vi "UI.vi"(0 "GUI":refnum<class "GUI Sensor Lib.lvclass">, 5 "error in (no error)":errorcluster) -> (14 "reference out":refnum<class "GUI Sensor Lib.lvclass">, 19 "error out":errorcluster)   [LabVIEW 2019, in "GUI Sensor Lib.lvclass"]
uses:
  GUI Sensor Lib.lvclass
  D:/GIT H4000/H4000/src/GUI_class/GUI.lvclass
  TypeDef/GUI AI Ranges.ctl
  TypeDef/AI_Data.ctl
  TypeDef/AI Statistics Data.ctl
  GUI_class/GUI.lvclass/GUI.ctl
  TypeDef/Scale Data.ctl
  TypeDef/AI_Data_Array.ctl
  SV_Wrap/SharedVariableWrapper.lvclass/SharedVariableWrapper.ctl
  TypeDef/CalibrationData.ctl
  TypeDef/GUI Setting Channel.ctl
  MessageAMC_class/MessageAMC.lvclass
  D:/GIT H4000/H4000/src/MessageInterface_class/MessageInterface.lvclass
  <vilib>/Utility/miscctls.llb/LVStringsAndValuesArrayTypeDef_U16.ctl
  3f3c674f-4e90-49b5-a3bd-8b60e7823021.vi
  423febd4-7e95-46d1-90fe-d3c0b325c46b.vi
  73d7f925-78bb-4209-8c05-97525a648225.vi
  GUI_class/Set Win State.vi
  GUI_class/protected/GetSheredData.vi
  3f3c674f-4e90-49b5-a3bd-8b60e7823021.vi/a0a37fc8-e280-45ed-9300-29015878ae2c.vi
  SV_Wrap/Write Var Info.vi
  SV_Wrap/Read Var Info.vi
  423febd4-7e95-46d1-90fe-d3c0b325c46b.vi/498ba6c8-7b3f-45b0-8939-59de8baaa4e4.vi
  SV_Wrap/Read connection str.vi
  <userlib>/_OpenG.lib/time/time.llb/Tick Count (ms)__ogtk.vi
  GUI_class/GUI.lvclass
  MessageInterface_class/MessageInterface.lvclass
  SV_Wrap/SharedVariableWrapper.lvclass
panel:
  out "element":T1 {"Stat Data"."scl mean 1Hz" format="%0.2f"; "Stat Data"."raw mean 1Hz" format="%0.2f"; "Stat Data"."scl mean" format="%0.2f"; "Stat Data"."raw mean" format="%0.2f"}
  in  "channel indx":T3(radio)
  in  "Edit scale":bool
  in  "Scales":i32(listbox) caption="Шкалы"
  in  "Remove scl":bool
  in  "Add scl":bool
  in  "channels":cluster{"name":string, "scale indx":u16}[](array[cluster])
  out "Gauge":dbl(knob) scale=0.0..10.0
  in  "manual enter raw":bool caption="Ввод  вручную"
  in  "Scaled":dbl caption="Калиброванное  значение"
  in  "Raw":dbl caption="Необработанное значение"
  in  "data":i32(listbox)
  in  "Remove":bool
  in  "Add":bool
  out "XY Graph - Dark":cluster{"X":dbl[], "Y":dbl[]}(graph) caption="Шкала"
  in  "AI Ranges":T4
  # "SCALED"
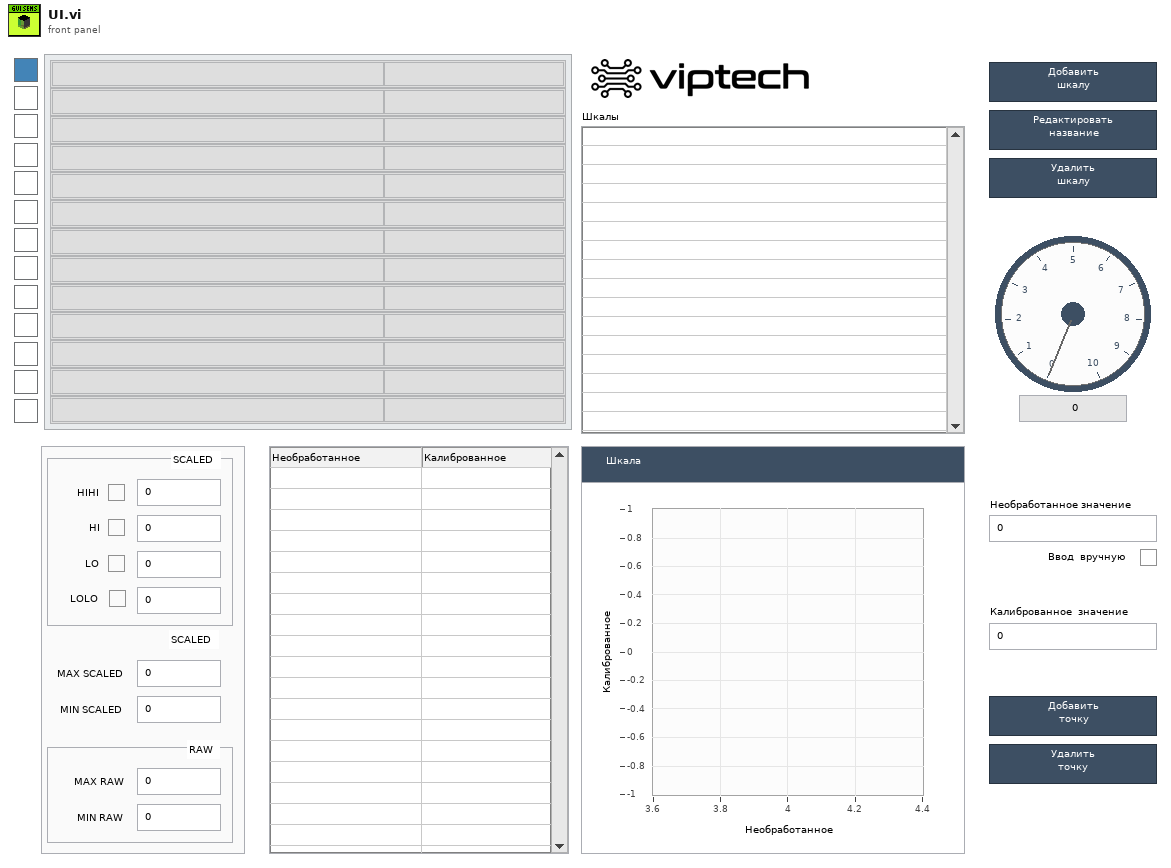
[diagram p1: front panel]
types:
  T1 = typedef "AI_Data.ctl" = cluster{"Stat Data":T2, "OutOfRangeMax":bool, "OutOfRangeMin":bool, "HIHI":bool, "HI":bool, "LO":bool, "LOLO":bool}
  T2 = typedef "AI Statistics Data.ctl" = cluster{"raw mean":dbl, "scl mean":dbl, "raw mean 1Hz":dbl, "scl mean 1Hz":dbl}
  T3 = enum32{"Item 0", "Item 1", "Item 2", "Item 3", "Item 4", "Item 5", "Item 6", "Item 7", "Item 8", "Item 9", "Item 10", "Item 11", "Item 12"}
  T4 = typedef "GUI AI Ranges.ctl" = cluster{"HI":bool, "HIHI":bool, "LO":bool, "LOLO":bool, "HIHI VAL":dbl, "HI VAL":dbl, "LO VAL":dbl, "LOLO VAL":dbl, "MAX RAW":dbl, "MIN RAW":dbl, "MAX SCALED":dbl, "MIN SCALED":dbl}
  T5 = typedef "Scale Data.ctl" = cluster{"index":i32, "Name":string, "X":dbl[], "Y":dbl[]}
  T6 = typedef "AI_Data_Array.ctl" = T1[]
  T7 = enum32{"Invalid", "Standard", "Closed", "Hidden", "Minimized", "Maximized"}
  T8 = enum32{"invalid app kind", "Development System", "Run Time System", "Student Edition", "Embedded LabVIEW", "Evaluation", "Custom"}
  T9 = typedef "CalibrationData.ctl" = cluster{"Channels":T10[], "Scales":T5[]}
  T10 = typedef "GUI Setting Channel.ctl" = cluster{"Name":string, "AI Ranges":T4, "ScaleIndex":u32}
  T11 = typedef "LVStringsAndValuesArrayTypeDef_U16.ctl" = cluster{"String":string, "Value":u16}[]
  T12 = cluster{"Core":cluster{"Current VI Reference":refnum<vi>, "Close Panel on Exit?":bool}, "CalibrationData":T9, "VAR":string, "valid data":bool, "amc":refnum<class "MessageAMC.lvclass">, "channel indx":enum32{"Item 0", "Item 1", "Item 2", "Item 3", "Item 4", "Item 5", "Item 6", "Item 7", "Item 8", "Item 9", "Item 10", "Item 11", "Item 12"}, "Scales ref":refnum<vi>, "scale indx ref":refnum<vi>}
  T13 = cluster{"Current VI Reference":refnum<vi>, "Close Panel on Exit?":bool}
  T14 = typedef "SharedVariableWrapper.lvclass/Config.ctl" = cluster{"connection str":string, "timeout":dbl, "ip":string}
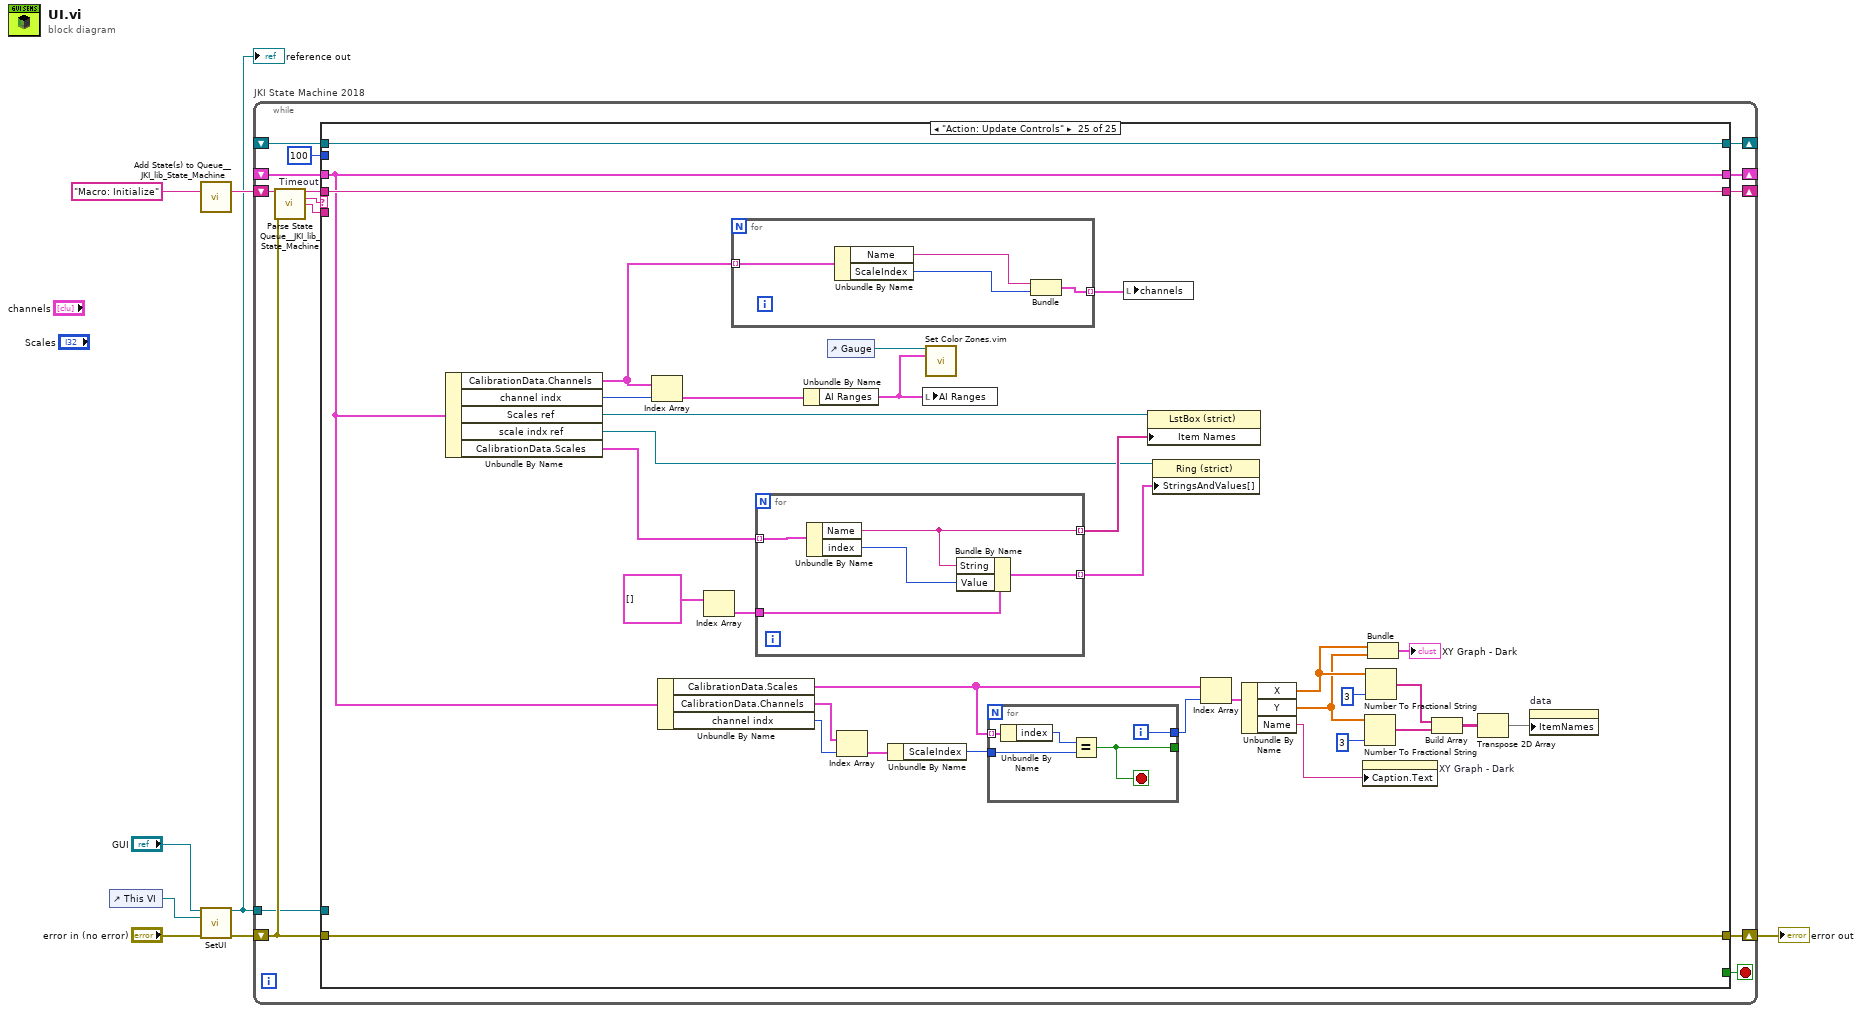
[diagram p0: block diagram]
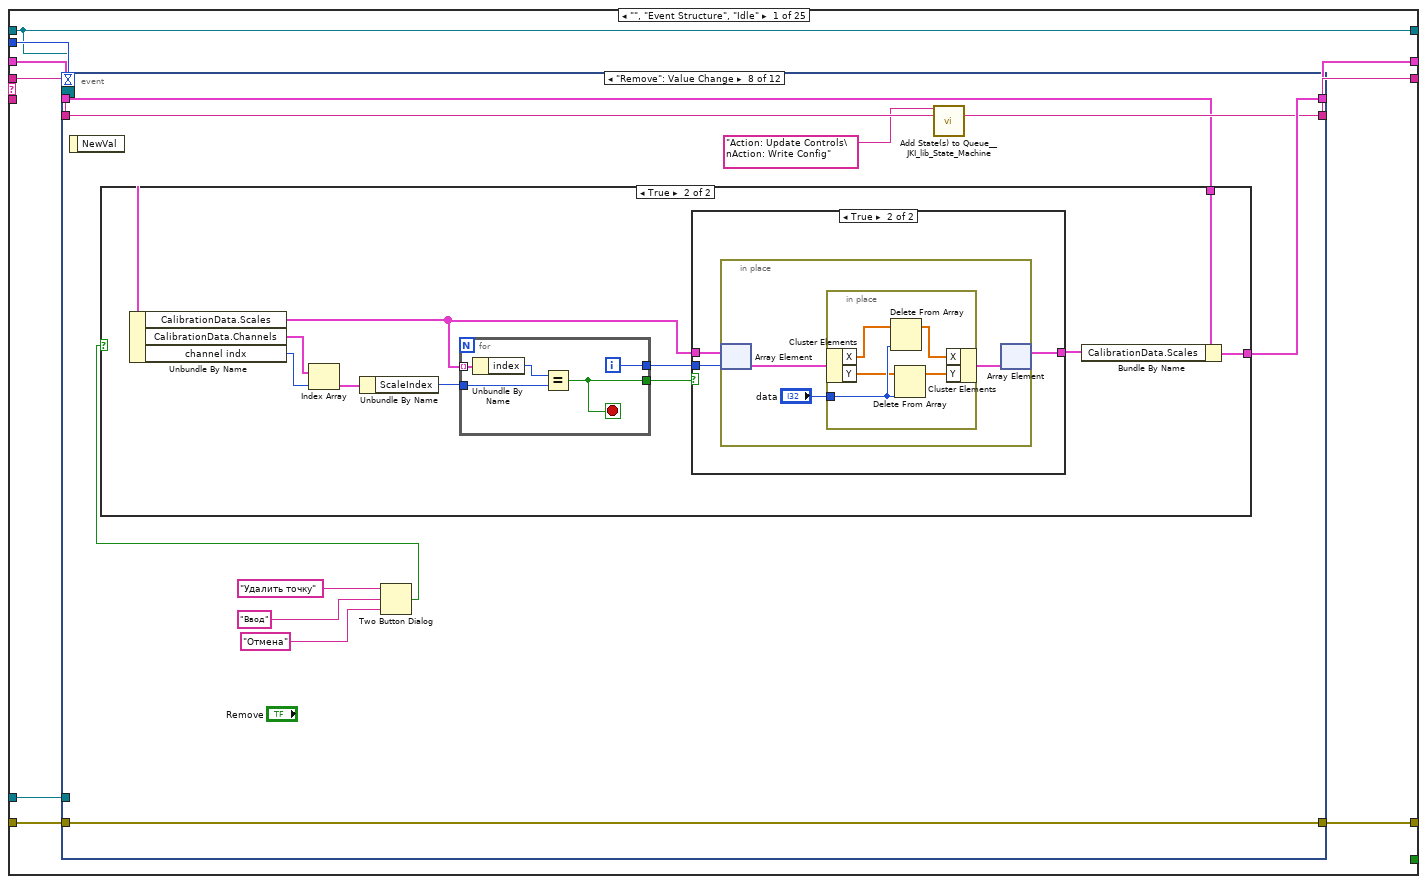
[diagram p2: hidden frame]
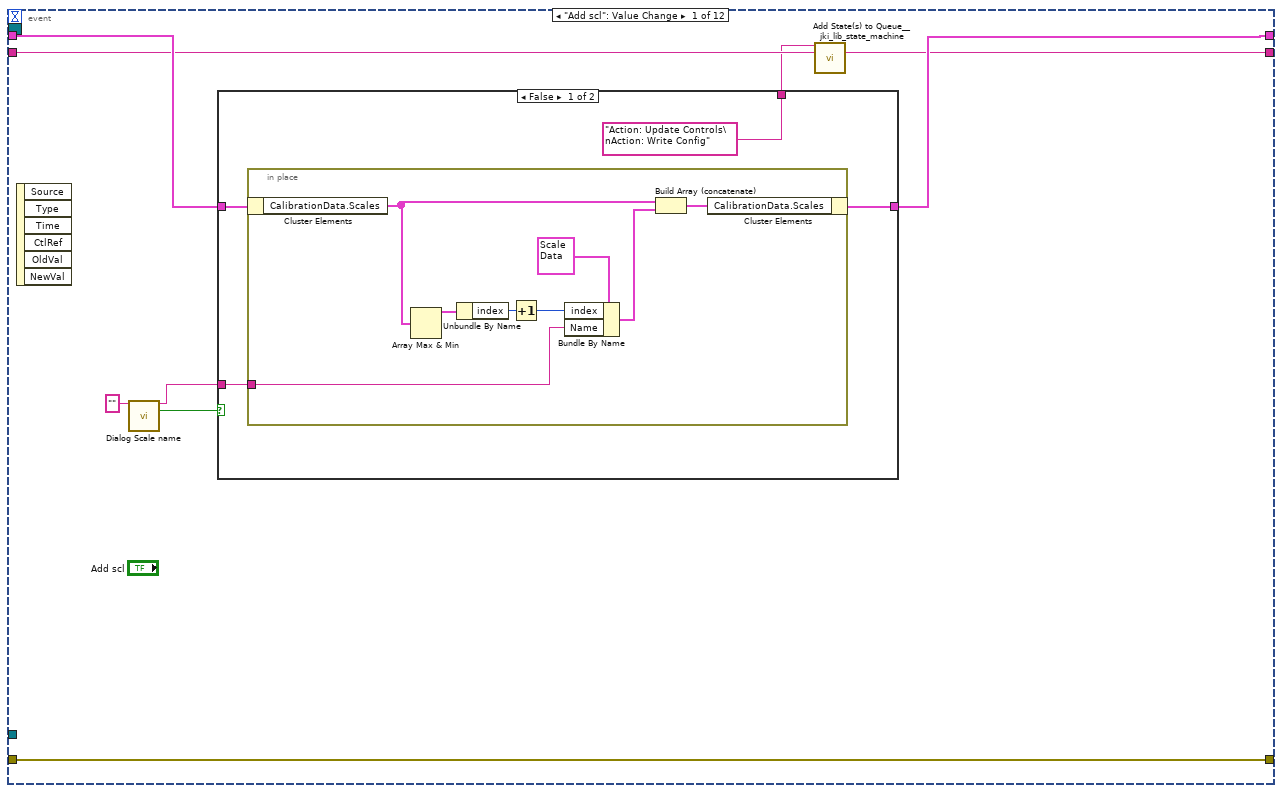
[diagram p3: hidden frame]
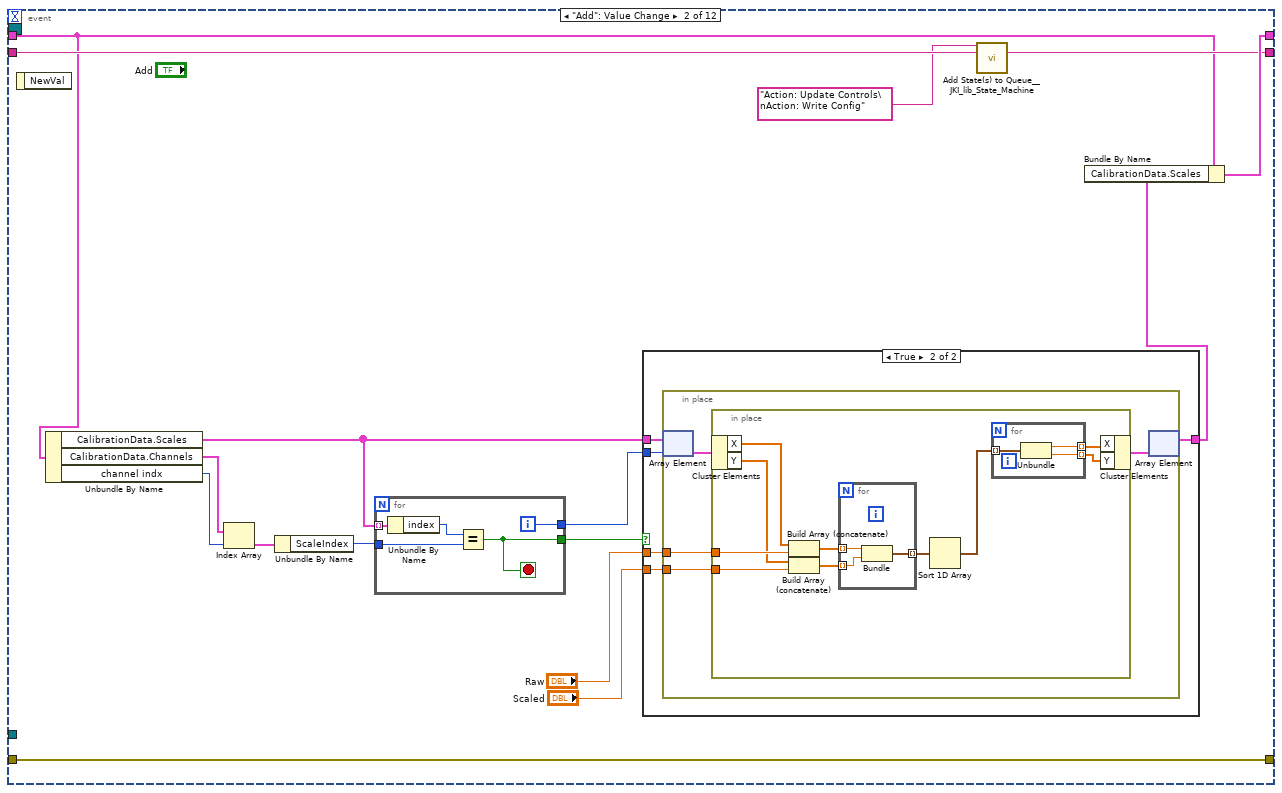
[diagram p5: hidden frame]
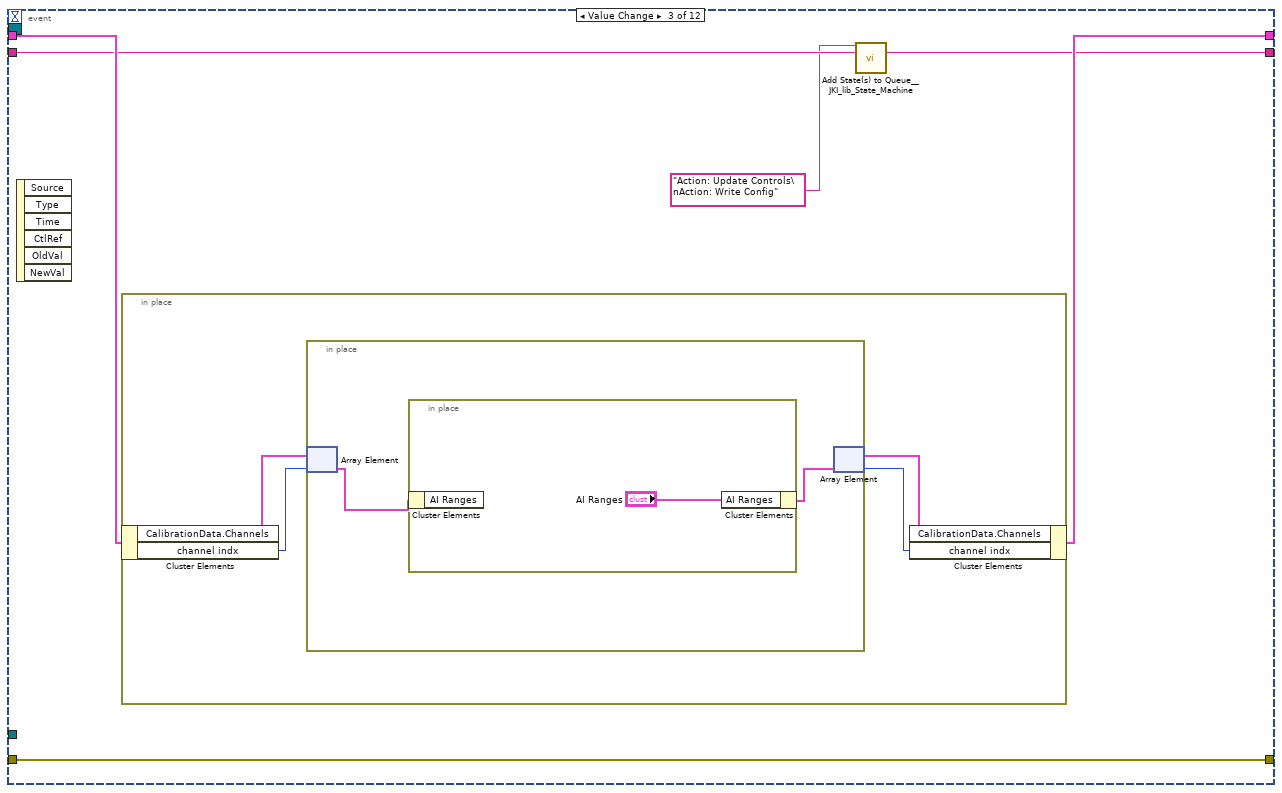
[diagram p7: hidden frame]
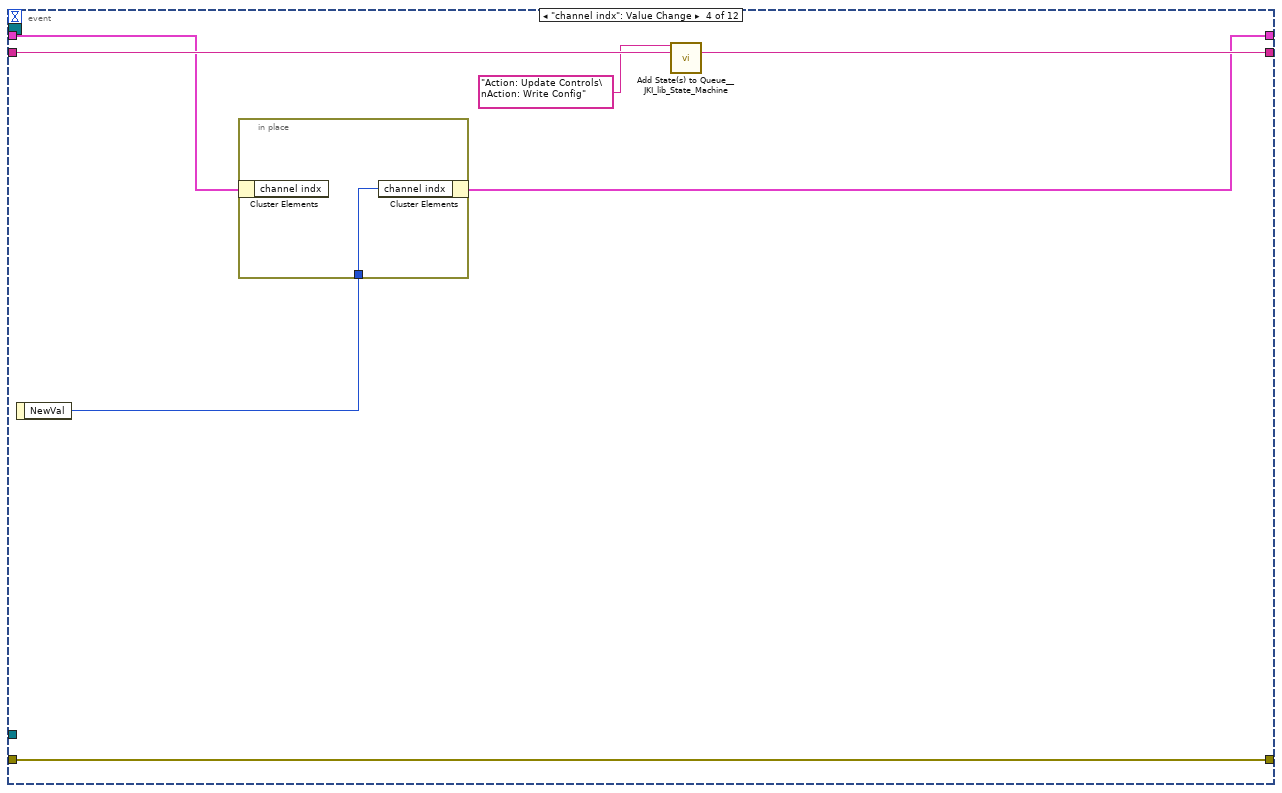
[diagram p8: hidden frame]
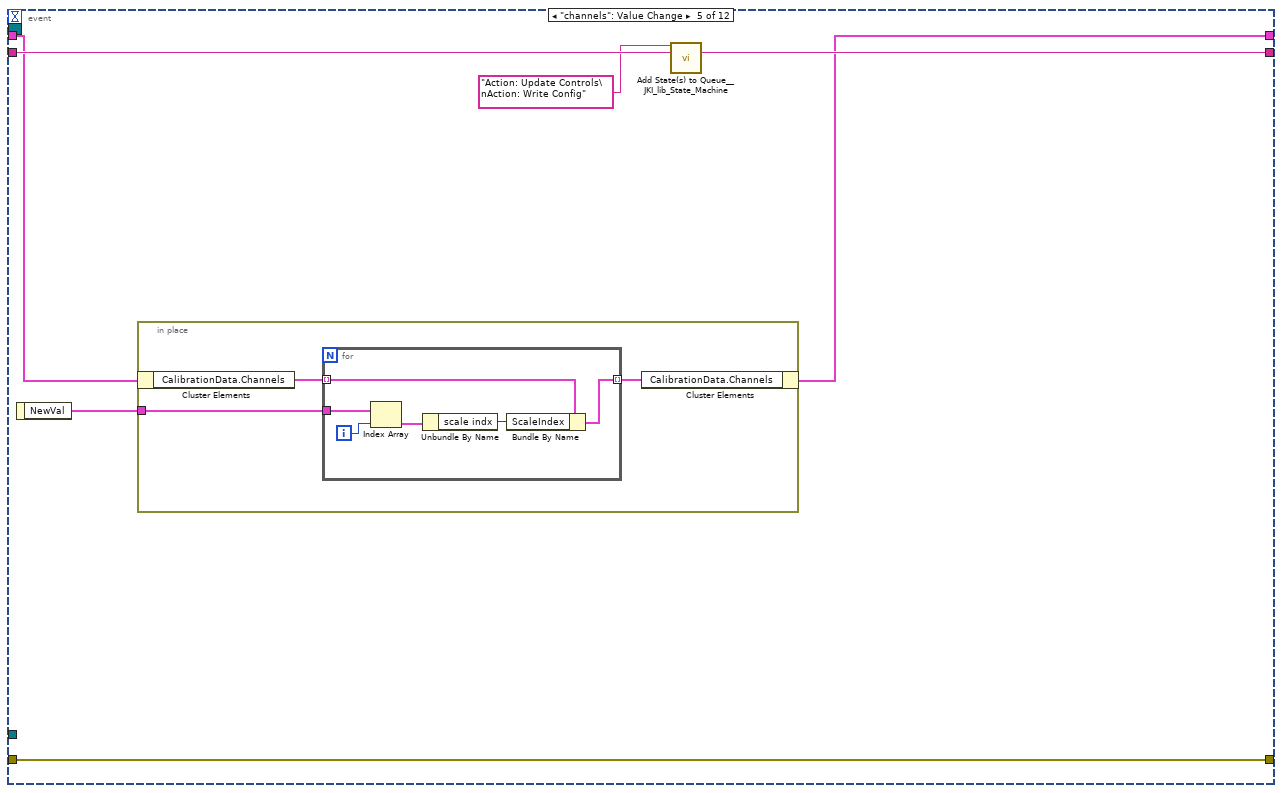
[diagram p9: hidden frame]
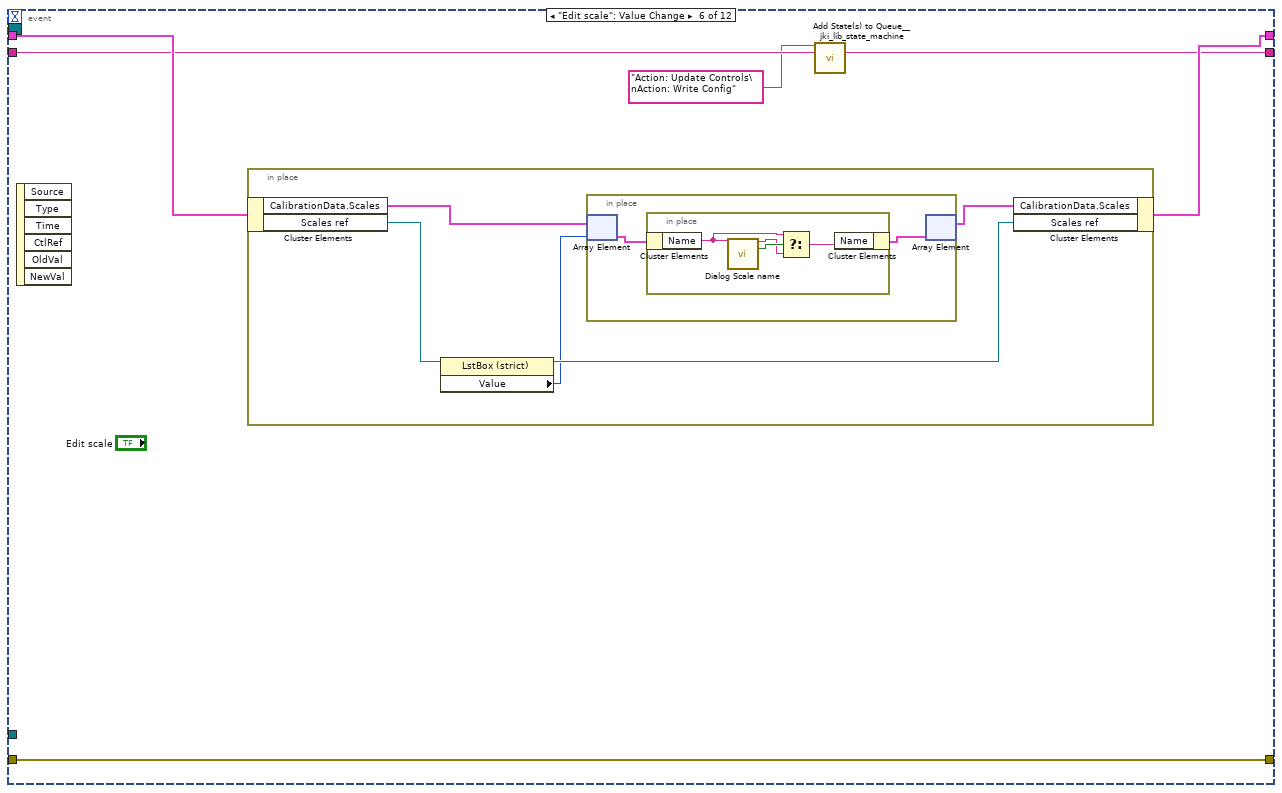
[diagram p10: hidden frame]
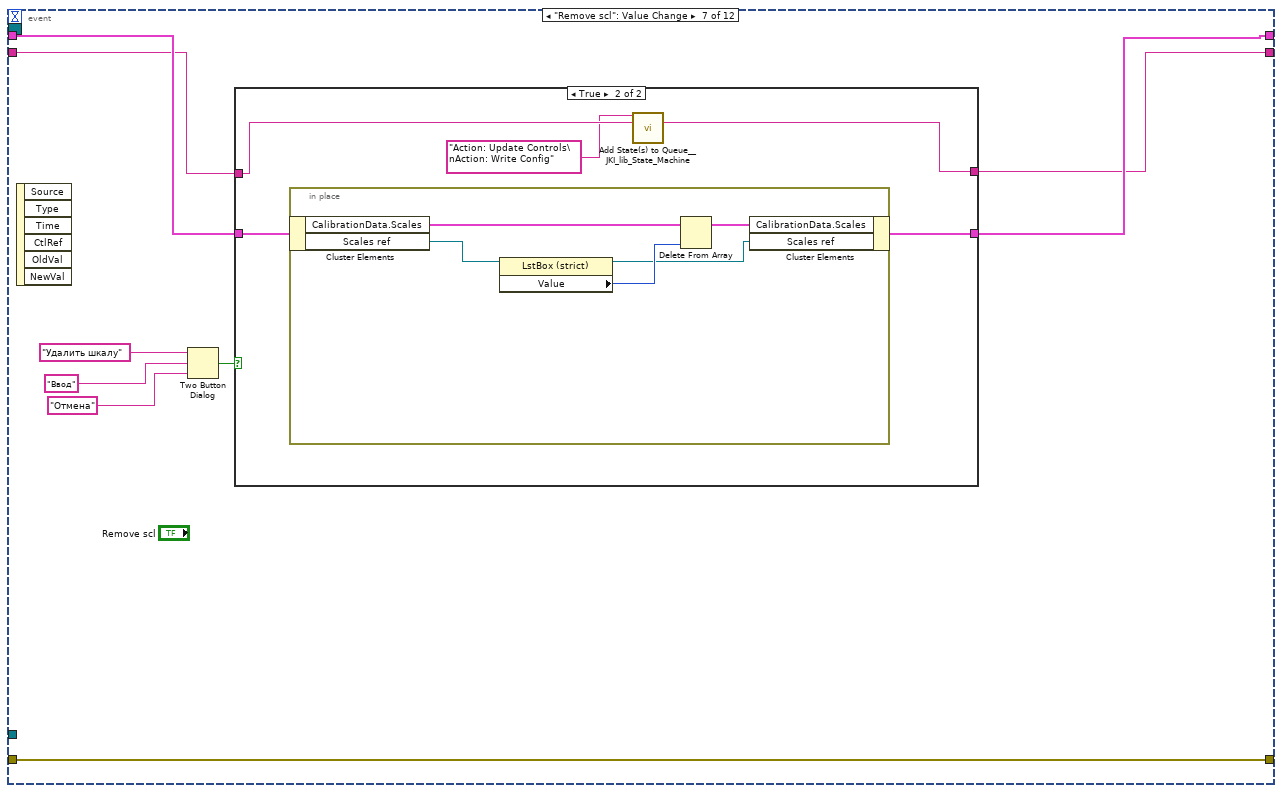
[diagram p11: hidden frame]
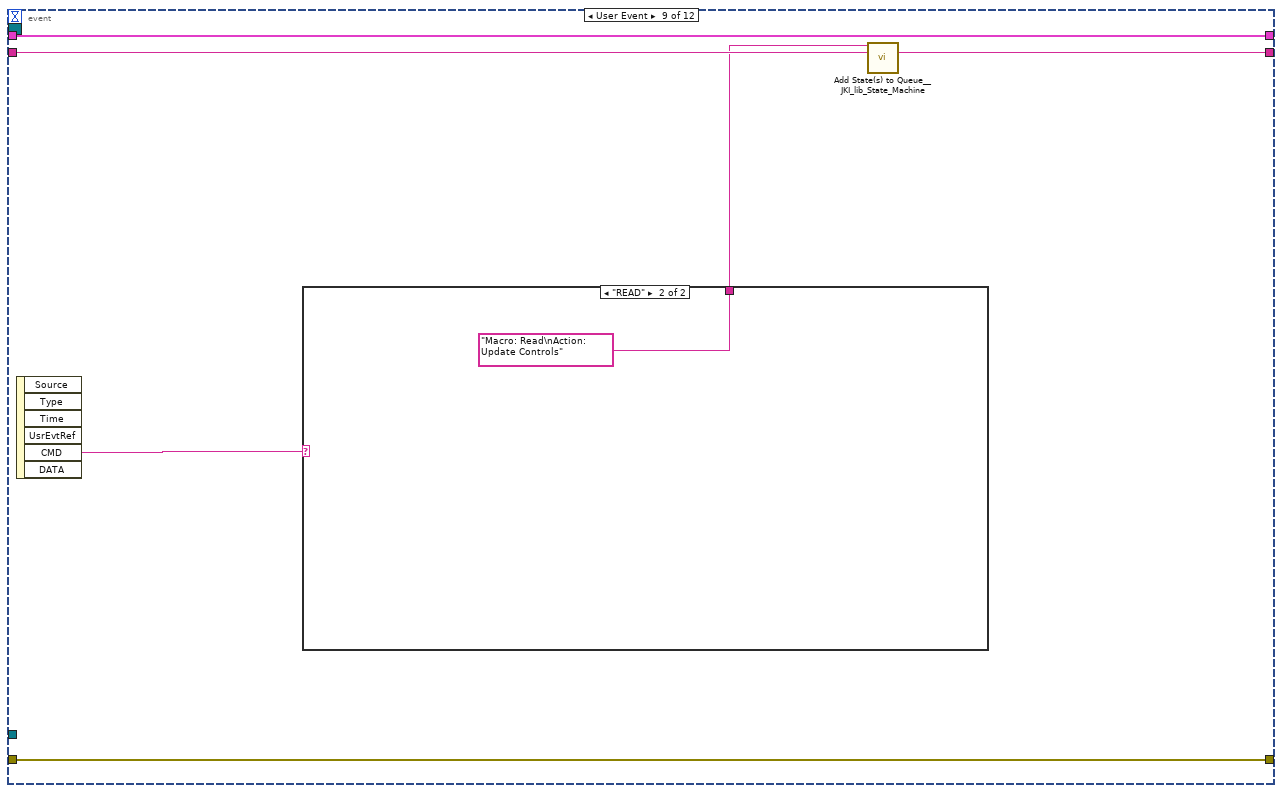
[diagram p15: hidden frame]
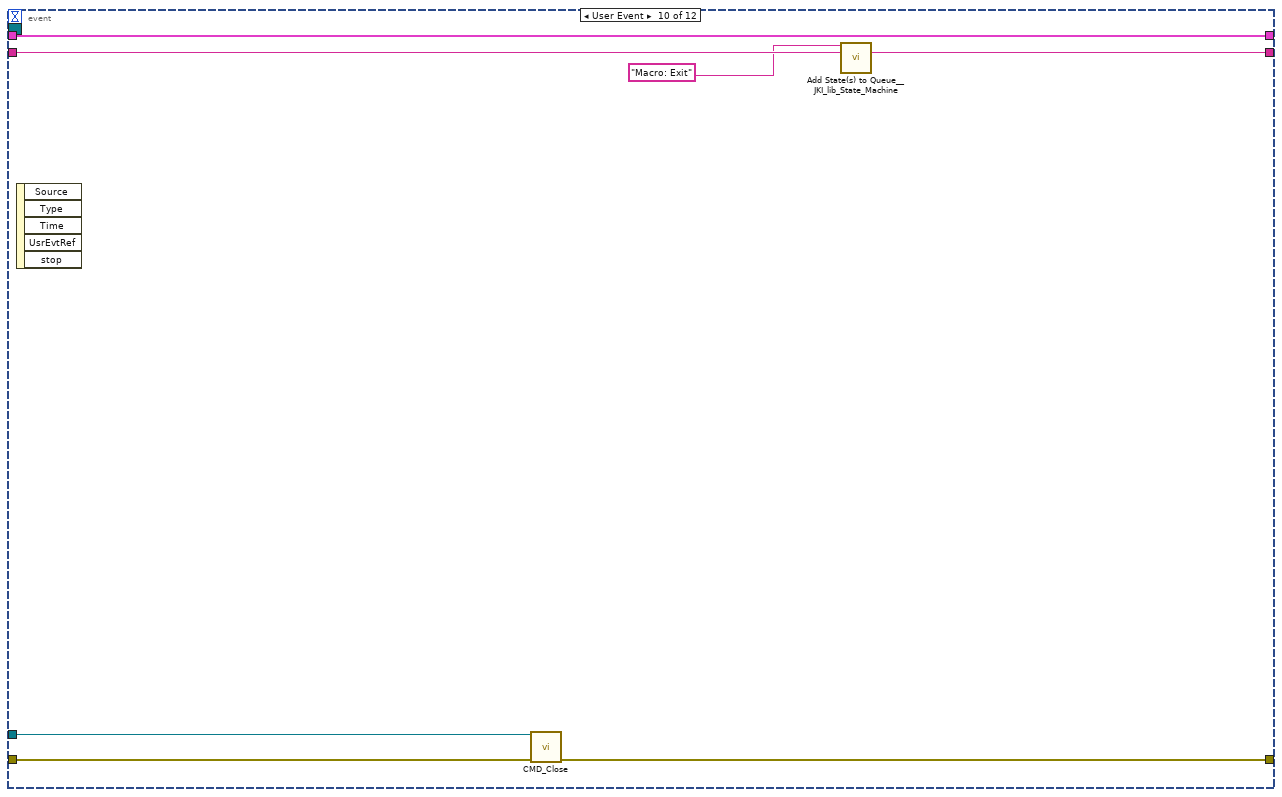
[diagram p17: hidden frame]
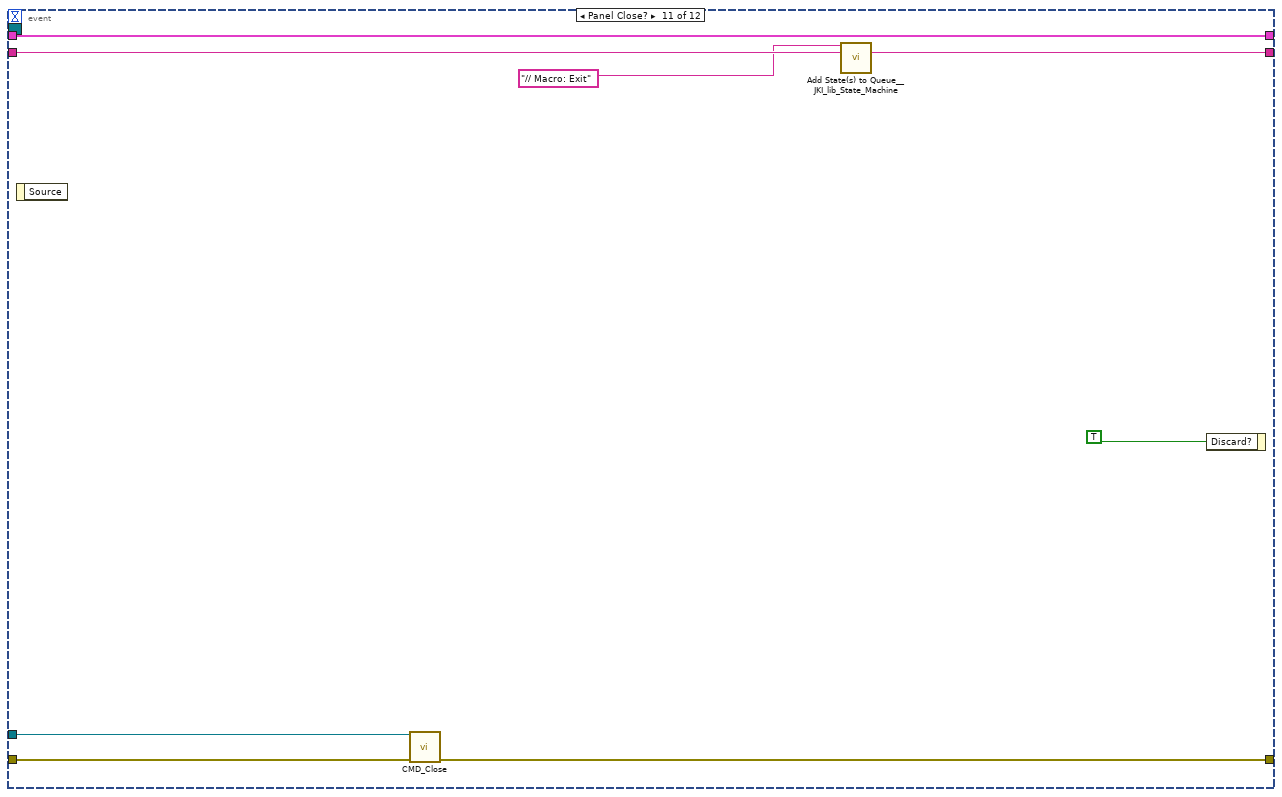
[diagram p18: hidden frame]
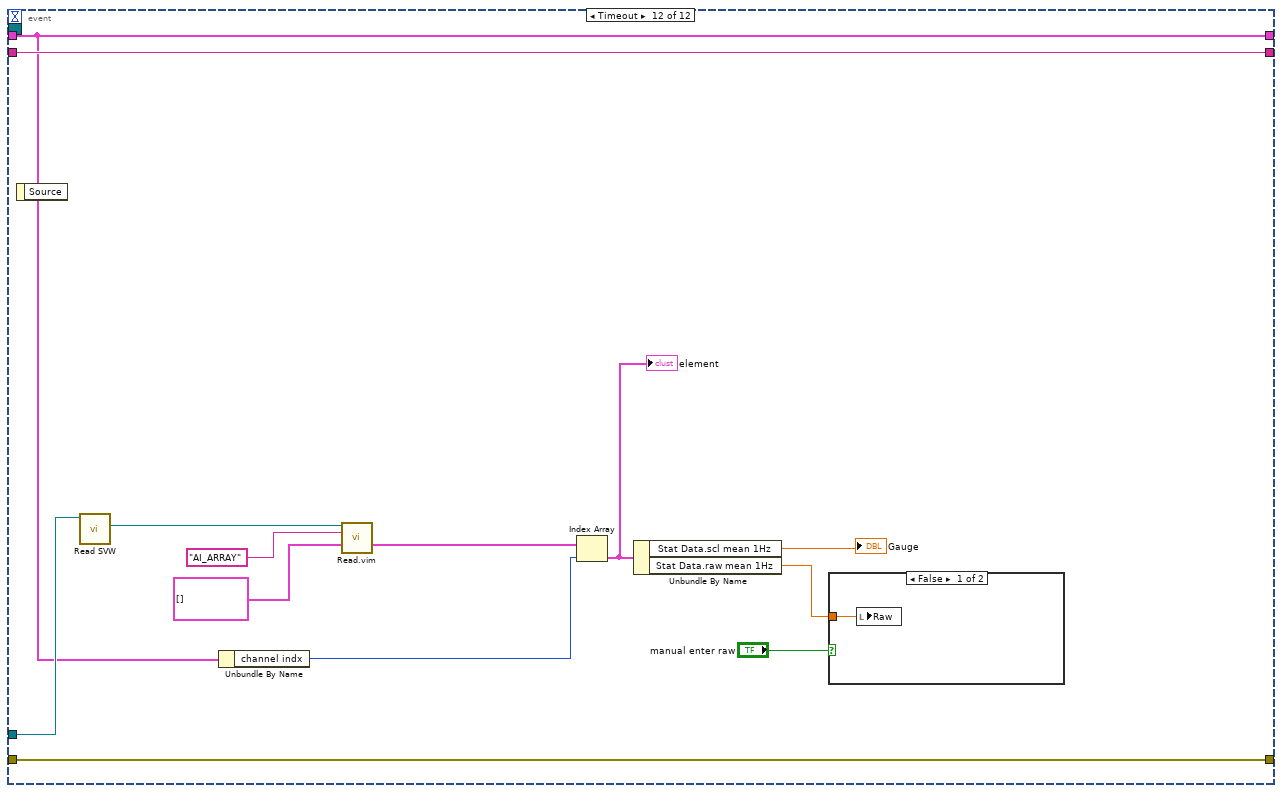
[diagram p19: hidden frame]
diagram:
  n1 = control-ref of="This VI"() -> (w3:refnum<vi>)
  n2 = call <vilib>:"Add State(s) to Queue__JKI_lib_State_Machine.vi"("State(s) in (\"\")"="Macro: Initialize") -> ("States Out"=w8:string)  [unwired: 14 in]
  n3 = call "SetUI.vi"("reference in"="GUI", "UI VI"=w3, "error in (no error)"="error in (no error)") -> ("reference out"=w1:refnum<class "GUI Sensor Lib.lvclass">, "error out"=w2:errorcluster)  [unwired: 11 in]
  "reference out" <- w1
  n4 = while "JKI State Machine 2018" {
    shift-right: [w15] -> _
    shift-left: _ -> [w14]
    shift-right: [w18] -> w6
    shift-left: w2 -> [w12]
    shift-right: [w17] -> _
    shift-left: w8 -> [w19]
    tunnel: w1 -> [w11]
    shift-right: [w10] -> _
    shift-left: _ -> [w9]
    stop <- w16 stop-if-true
    w13 = 100  # Timeout
    n5 = call <vilib>:"Parse State Queue__JKI_lib_State_Machine.vi"("State Queue"=w19, "Error In (no error)"=w12) -> ("Remaining States"=w21:string, "Current State"=w22:string, "Arguments"=w20:string)  [unwired: 11 in]
    n6 = case shown="\"Action: Update Controls\"" w22 {
      selector: w22 -> [_ _ w256 _ _ _ _ _ _ _ _ _ _ _ _ _ _ _ _ _ _ _ _ _ _]
      tunnel: w21 -> [w31 w254 w260 w280 w287 w293 w298 w313 w320 w325 w333 w339 w344 w348 w355 w367 w437 w443 w449 w455 w467 w471 w475 w500 w545]
      tunnel: w20 -> [_ _ _ _ _ _ _ _ _ _ _ _ _ _ w350 w361 _ _ _ _ _ _ _ _ _]
      tunnel: w14 -> [w29 w251 w258 w273 w284 w291 w295 _ w315 w322 w332 w337 w341 w347 w353 w363 w434 w440 w446 w452 w464 w469 w481 w497 w523]
      tunnel: [w28 w252 w262 w277 errorcluster {"status"=FALSE, "code"=0, "source"=""} ("error out") w290 w296 w302 w316 w323 w330 w334 w342 w346 w351 w364 w435 w441 w447 w453 w465 w470 w472 w494 w547] -> w18
      tunnel: w12 -> [w27 w252 w261 w277 w283 w290 w296 w303 w317 w323 w329 w335 w342 w346 w352 w365 w435 w441 w447 w453 w465 w470 w477 w494 w547]
      tunnel: [w30 w253 w259 w279 w286 w292 w297 w313 w319 w324 w333 w338 w343 w348 w354 w366 w436 w442 w448 w454 w466 w471 w476 w500 w545] -> w17
      tunnel: [_ _ _ _ _ TRUE _ _ _ _ _ _ _ _ _ _ _ _ _ _ _ _ _ _ _] -> w16
      tunnel: [w26 w251 w258 w278 w284 w291 w295 w312 w315 w322 w332 w337 w341 w347 w353 w363 w434 w440 w446 w452 w464 w469 w483 w497 w523] -> w15
      tunnel: w13 -> [w25 _ _ _ _ _ _ _ _ _ _ _ _ _ _ _ _ _ _ _ _ _ _ _ _]
      tunnel: w11 -> [w24 _ _ _ _ _ _ _ _ _ w328 _ _ _ _ _ _ _ _ _ _ _ w479 w496 _]
      tunnel: [w23 w250 w255 w267 w281 w288 w294 w310 w314 w321 w331 w336 w340 w345 w349 w360 w433 w438 w444 w450 w457 w468 w484 w499 w546] -> w10
      tunnel: w9 -> [w23 w250 w255 w267 w281 w288 w294 w310 w314 w321 _ w336 w340 w345 w349 w360 w433 w438 w444 w450 w457 w468 w484 w499 w546]
      frame "", "Event Structure", "Idle" {
        n7 = event shown="[7] \"Remove\": Value Change" {
          selector: w23 -> [_ _ _ _ _ _ _ _ _ _ _ _]
          dyn-events: _ -> [_ _ _ _ _ _ _ _ _ _ _ _]
          timeout: w25 -> [_ _ _ _ _ _ _ _ _ _ _ _]
          tunnel: w31 -> [w33 w66 w102 w118 w126 w139 w159 w182 w215 w227 w235 w248]
          tunnel: [w34 w67 w103 w119 w127 w140 w160 w183 w216 w226 w234 w248] -> w30
          tunnel: w29 -> [w39 w58 w105 w116 w122 w142 w162 w180 w218 w225 w233 w239]
          tunnel: [w40 w69 w106 w120 w128 w143 w163 w185 w219 w221 w228 w247] -> w28
          tunnel: w27 -> [w40 w69 w106 w120 w128 w143 w163 w185 w219 w222 w229 w247]
          tunnel: [w38 w68 w104 w115 w124 w141 w161 w184 w218 w225 w233 w239] -> w26
          tunnel: w24 -> [_ _ _ _ _ _ _ _ _ w223 w230 w244]
          event "Add scl": Value Change {
            n8 = event-data() -> ()  [unwired: 1 in, 6 out]
            n9 = call "Dialog Scale name.vi"("name in"="") -> ("name out"=w35:string, "canceled"=w36:bool)  [unwired: 13 in]
            n10 = case shown="False" w36 {
              tunnel: w39 -> [w44 w53]
              tunnel: [w43 w53] -> w38
              tunnel: w35 -> [w42 _]
              tunnel: ["Action: Update Controls\nAction: Write Config" ("State(s) in Front (\"\")") _] -> w32
              frame False {
                n11 = in-place {
                  in-place-border: w42 -> [w45]
                  n12 = in-place-cluster #1(w44) -> ("CalibrationData.Scales"=w49:T5[])
                  n13 = Array Max & Min(array=w49) -> (max value=w51:T5)  [unwired: 3 out]
                  n14 = Unbundle By Name(w51) -> ("index"=w50:i32)
                  n15 = Increment(x=w50) -> (x+1=w46:i32)
                  n16 = Bundle By Name(cluster=T5 {"index"=0, "Name"="", "X"=[4.0, 20.0], "Y"=[4.0, 20.0]} ("value"), "index"=w46, "Name"=w45) -> (w48:T5)
                  n17 = Build Array (concatenate)(w49, w48) -> (w47:T5[])
                  n18 = in-place-cluster #1("CalibrationData.Scales"=w47) -> (w43:T12)
                }
              }
              frame True {
              }
            }
            n19 = call <vilib>:"Add State(s) to Queue__jki_lib_state_machine.vi"("State(s) in Front (\"\")"=w32, "State(s) in (\"\")"=w33) -> ("States Out"=w34:string)  [unwired: 13 in]
          }
          event "Add": Value Change {
            n20 = event-data() -> ()  [unwired: 1 in, 1 out]
            n21 = Unbundle By Name(w58) -> ("CalibrationData.Scales"=w57:T5[], "CalibrationData.Channels"=w64:T10[], "channel indx"=w61:T3)
            n22 = Index Array(array=w64, index=w61) -> (element=w60:T10)
            n23 = Unbundle By Name(w60) -> ("ScaleIndex"=w59:u32)
            n24 = for {
              tunnel: w57 -> [w100] mode=indexing
              tunnel: w59 -> [w99]
              tunnel: [w97] -> w54
              tunnel: [w96] -> w56
              i -> [w96]
              stop <- w97 stop-if-true
              n25 = Unbundle By Name(w100) -> ("index"=w98:i32)
              n26 = Equal?(x=w98, y=w99) -> (x = y?=w97:bool)
            }
            n27 = case shown="True" w54 {
              tunnel: "Scaled" -> [_ w75]
              tunnel: "Raw" -> [_ w74]
              tunnel: w57 -> [w70 w73]
              tunnel: w56 -> [_ w72]
              tunnel: [w70 w71] -> w55
              frame False {
              }
              frame True {
                n28 = in-place {
                  in-place-border: w75 -> [w79]
                  in-place-border: w74 -> [w78]
                  n29 = in-place-array #2(w73, w72) -> (w77:T5)
                  n30 = in-place {
                    in-place-border: w79 -> [w89]
                    in-place-border: w78 -> [w88]
                    n31 = in-place-cluster #3(w77) -> ("X"=w83:dbl[], "Y"=w82:dbl[])
                    n32 = Build Array (concatenate)(w83, w88) -> (w85:dbl[])
                    n33 = Build Array (concatenate)(w82, w89) -> (w84:dbl[])
                    n34 = for {
                      tunnel: w85 -> [w95] mode=indexing
                      tunnel: w84 -> [w94] mode=indexing
                      tunnel: [w93] -> w86 mode=indexing
                      n35 = Bundle("Raw"=w95, "Scaled"=w94) -> (w93:cluster{"Raw":dbl, "Scaled":dbl})  [unwired: 1 in]
                    }
                    n36 = Sort 1D Array(array=w86) -> (sorted array=w87:cluster{"Raw":dbl, "Scaled":dbl}[])
                    n37 = for {
                      tunnel: w87 -> [w92] mode=indexing
                      tunnel: [w91] -> w81 mode=indexing
                      tunnel: [w90] -> w80 mode=indexing
                      n38 = Unbundle(w92) -> ("Raw"=w91:dbl, "Scaled"=w90:dbl)
                    }
                    n39 = in-place-cluster #3("X"=w81, "Y"=w80) -> (w76:T5)
                  }
                  n40 = in-place-array #2(w76) -> (w71:T5[])  [unwired: 1 out]
                }
              }
            }
            n41 = call <vilib>:"Add State(s) to Queue__JKI_lib_State_Machine.vi"("State(s) in Front (\"\")"="Action: Update Controls\nAction: Write Config" ("State(s) in Front (\"\")"), "State(s) in (\"\")"=w66) -> ("States Out"=w67:string)  [unwired: 13 in]
            n42 = Bundle By Name(cluster=w58, "CalibrationData.Scales"=w55) -> (w68:T12)
          }
          event Value Change {
            n43 = event-data() -> ()  [unwired: 1 in, 6 out]
            n44 = in-place {
              n45 = in-place-cluster #4(w105) -> ("CalibrationData.Channels"=w110:T10[], "channel indx"=w108:T3)
              n46 = in-place {
                n47 = in-place-array #5(w110, w108) -> (w112:T10)
                n48 = in-place {
                  n49 = in-place-cluster #6(w112) -> ()  [unwired: 1 out]
                  n50 = in-place-cluster #6("AI Ranges"="AI Ranges") -> (w111:T10)
                }
                n51 = in-place-array #5(w111) -> (w109:T10[], w107:i32)
              }
              n52 = in-place-cluster #4("CalibrationData.Channels"=w109, "channel indx"=w107) -> (w104:T12)
            }
            n53 = call <vilib>:"Add State(s) to Queue__JKI_lib_State_Machine.vi"("State(s) in Front (\"\")"="Action: Update Controls\nAction: Write Config" ("State(s) in Front (\"\")"), "State(s) in (\"\")"=w102) -> ("States Out"=w103:string)  [unwired: 13 in]
          }
          event "channel indx": Value Change {
            n54 = event-data() -> ("NewVal"=w114:T3)  [unwired: 1 in]
            n55 = in-place {
              in-place-border: w114 -> [w121]
              n56 = in-place-cluster #7(w116) -> ()  [unwired: 1 out]
              n57 = in-place-cluster #7("channel indx"=w121) -> (w115:T12)
            }
            n58 = call <vilib>:"Add State(s) to Queue__JKI_lib_State_Machine.vi"("State(s) in Front (\"\")"="Action: Update Controls\nAction: Write Config" ("State(s) in Front (\"\")"), "State(s) in (\"\")"=w118) -> ("States Out"=w119:string)  [unwired: 13 in]
          }
          event "channels": Value Change {
            n59 = event-data() -> ("NewVal"=w123:cluster{"name":string, "scale indx":u16}[])  [unwired: 1 in]
            n60 = in-place {
              in-place-border: w123 -> [w129]
              n61 = in-place-cluster #8(w122) -> ("CalibrationData.Channels"=w131:T10[])
              n62 = for {
                tunnel: w131 -> [w137] mode=indexing
                tunnel: [w133] -> w130 mode=indexing
                tunnel: w129 -> [w136]
                i -> [w135]
                n63 = Index Array(array=w136, index=w135) -> (element=w134:cluster{"name":string, "scale indx":u16})
                n64 = Unbundle By Name(w134) -> ("scale indx"=w132:u16)
                n65 = Bundle By Name(cluster=w137, "ScaleIndex"=w132) -> (w133:T10)
              }
              n66 = in-place-cluster #8("CalibrationData.Channels"=w130) -> (w124:T12)
            }
            n67 = call <vilib>:"Add State(s) to Queue__JKI_lib_State_Machine.vi"("State(s) in Front (\"\")"="Action: Update Controls\nAction: Write Config" ("State(s) in Front (\"\")"), "State(s) in (\"\")"=w126) -> ("States Out"=w127:string)  [unwired: 13 in]
          }
          event "Edit scale": Value Change {
            n68 = event-data() -> ()  [unwired: 1 in, 6 out]
            n69 = in-place {
              n70 = in-place-cluster #9(w142) -> ("CalibrationData.Scales"=w146:T5[], "Scales ref"=w148:refnum<vi>)
              n71 = property class="LstBox (strict)"(reference=w148) -> (reference out=w147:refnum<vi>, "Value"=w145:i32)  [unwired: 1 in, 1 out]
              n72 = in-place {
                n73 = in-place-array #10(w146, w145) -> (w150:T5)
                n74 = in-place {
                  n75 = in-place-cluster #11(w150) -> ("Name"=w153:string)
                  n76 = call "Dialog Scale name.vi"("name in"=w153) -> ("name out"=w152:string, "canceled"=w154:bool)  [unwired: 13 in]
                  n77 = Select(t=w153, s=w154, f=w152) -> (s? t:f=w151:string)
                  n78 = in-place-cluster #11("Name"=w151) -> (w149:T5)
                }
                n79 = in-place-array #10(w149) -> (w144:T5[])  [unwired: 1 out]
              }
              n80 = in-place-cluster #9("CalibrationData.Scales"=w144, "Scales ref"=w147) -> (w141:T12)
            }
            n81 = call <vilib>:"Add State(s) to Queue__jki_lib_state_machine.vi"("State(s) in Front (\"\")"="Action: Update Controls\nAction: Write Config" ("State(s) in Front (\"\")"), "State(s) in (\"\")"=w139) -> ("States Out"=w140:string)  [unwired: 13 in]
          }
          event "Remove scl": Value Change {
            n82 = event-data() -> ()  [unwired: 1 in, 6 out]
            n83 = Two Button Dialog(message="Удалить шкалу", 1:"Отмена" ("F button name (\"Cancel\")"), 2:"Ввод" ("T button name (\"OK\")")) -> (T button?=w155:bool)
            n84 = case shown="True" w155 {
              tunnel: w162 -> [w165 w170]
              tunnel: [w165 w169] -> w161
              tunnel: [w164 w168] -> w160
              tunnel: w159 -> [w164 w167]
              frame False {
              }
              frame True {
                n85 = in-place {
                  n86 = in-place-cluster #12(w170) -> ("CalibrationData.Scales"=w175:T5[], "Scales ref"=w173:refnum<vi>)
                  n87 = property class="LstBox (strict)"(reference=w173) -> (reference out=w171:refnum<vi>, "Value"=w172:i32)  [unwired: 1 in, 1 out]
                  n88 = Delete From Array(array=w175, index=w172) -> (array with subset deleted=w174:T5[])  [unwired: 1 in, 1 out]
                  n89 = in-place-cluster #12("CalibrationData.Scales"=w174, "Scales ref"=w171) -> (w169:T12)
                }
                n90 = call <vilib>:"Add State(s) to Queue__JKI_lib_State_Machine.vi"("State(s) in Front (\"\")"="Action: Update Controls\nAction: Write Config" ("State(s) in Front (\"\")"), "State(s) in (\"\")"=w167) -> ("States Out"=w168:string)  [unwired: 13 in]
              }
            }
          }
          event "Remove": Value Change {
            n91 = event-data() -> ()  [unwired: 1 in, 1 out]
            n92 = Two Button Dialog(message="Удалить точку", 1:"Отмена" ("F button name (\"Cancel\")"), 2:"Ввод" ("T button name (\"OK\")")) -> (T button?=w176:bool)
            n93 = case shown="True" w176 {
              tunnel: [w186 w196] -> w184
              tunnel: w180 -> [w186 w191]
              frame False {
              }
              frame True {
                n94 = Unbundle By Name(w191) -> ("CalibrationData.Scales"=w189:T5[], "CalibrationData.Channels"=w195:T10[], "channel indx"=w194:T3)
                n95 = Index Array(array=w195, index=w194) -> (element=w193:T10)
                n96 = Unbundle By Name(w193) -> ("ScaleIndex"=w192:u32)
                n97 = for {
                  tunnel: w189 -> [w213] mode=indexing
                  tunnel: w192 -> [w212]
                  tunnel: [w210] -> w187
                  tunnel: [w209] -> w190
                  i -> [w209]
                  stop <- w210 stop-if-true
                  n98 = Unbundle By Name(w213) -> ("index"=w211:i32)
                  n99 = Equal?(x=w211, y=w212) -> (x = y?=w210:bool)
                }
                n100 = case shown="True" w187 {
                  tunnel: w190 -> [_ w200]
                  tunnel: w189 -> [w197 w199]
                  tunnel: [w197 w198] -> w188
                  frame False {
                  }
                  frame True {
                    n101 = in-place {
                      n102 = in-place-array #13(w199, w200) -> (w202:T5)
                      n103 = in-place {
                        in-place-border: "data" -> [w208]
                        n104 = in-place-cluster #14(w202) -> ("X"=w207:dbl[], "Y"=w206:dbl[])
                        n105 = Delete From Array(array=w207, index=w208) -> (array with subset deleted=w204:dbl[])  [unwired: 1 in, 1 out]
                        n106 = Delete From Array(array=w206, index=w208) -> (array with subset deleted=w205:dbl[])  [unwired: 1 in, 1 out]
                        n107 = in-place-cluster #14("X"=w204, "Y"=w205) -> (w201:T5)
                      }
                      n108 = in-place-array #13(w201) -> (w198:T5[])  [unwired: 1 out]
                    }
                  }
                }
                n109 = Bundle By Name(cluster=w191, "CalibrationData.Scales"=w188) -> (w196:T12)
              }
            }
            n110 = call <vilib>:"Add State(s) to Queue__JKI_lib_State_Machine.vi"("State(s) in Front (\"\")"="Action: Update Controls\nAction: Write Config" ("State(s) in Front (\"\")"), "State(s) in (\"\")"=w182) -> ("States Out"=w183:string)  [unwired: 13 in]
          }
          event User Event {
            n111 = event-data() -> ("CMD"=w217:string)  [unwired: 1 in, 5 out]
            n112 = case shown="\"READ\"" w217 {
              tunnel: [_ "Macro: Read\nAction: Update Controls" ("State(s) in Front (\"\")")] -> w214
              frame Default {
              }
              frame "READ" {
              }
            }
            n113 = call <vilib>:"Add State(s) to Queue__JKI_lib_State_Machine.vi"("State(s) in Front (\"\")"=w214, "State(s) in (\"\")"=w215) -> ("States Out"=w216:string)  [unwired: 13 in]
          }
          event User Event {
            n114 = event-data() -> ()  [unwired: 1 in, 5 out]
            n115 = call "CMD_Close.vi"("reference in"=w223, "error in (no error)"=w222) -> ("error out"=w221:errorcluster)  [unwired: 12 in, 1 out]
            n116 = call <vilib>:"Add State(s) to Queue__JKI_lib_State_Machine.vi"("State(s) in Front (\"\")"="Macro: Exit", "State(s) in (\"\")"=w227) -> ("States Out"=w226:string)  [unwired: 13 in]
          }
          event Panel Close? {
            n117 = event-data() -> ()  [unwired: 1 in, 1 out]
            n118 = call "CMD_Close.vi"("reference in"=w230, "error in (no error)"=w229) -> ("error out"=w228:errorcluster)  [unwired: 12 in, 1 out]
            n119 = call <vilib>:"Add State(s) to Queue__JKI_lib_State_Machine.vi"("State(s) in Front (\"\")"="// Macro: Exit", "State(s) in (\"\")"=w235) -> ("States Out"=w234:string)  [unwired: 13 in]
            n120 = event-data("Discard?"=TRUE) -> ()  [unwired: 1 in, 1 out]
          }
          event Timeout {
            n121 = event-data() -> ()  [unwired: 1 in, 1 out]
            n122 = call "Read SVW.vi"("GUI in"=w244) -> ("SharedVariableWrapper.lvclass"=w243:refnum<class "SharedVariableWrapper.lvclass">)  [unwired: 10 in]
            n123 = Unbundle By Name(w239) -> ("channel indx"=w237:T3)
            n124 = call "Read.vim"("SharedVariableWrapper in"=w243, "name"="AI_ARRAY", "DataType"=T6 [] ("AI_Data_Array")) -> ("data out"=w238:T6)  [unwired: 6 in, 6 out]
            n125 = Index Array(array=w238, index=w237) -> (element=w236:T1)
            "element" <- w236
            n126 = Unbundle By Name(w236) -> ("Stat Data.scl mean 1Hz"=→"Gauge":dbl, "Stat Data.raw mean 1Hz"=w241:dbl)
            n127 = case shown="False" "manual enter raw" {
              tunnel: w241 -> [w249 _]
              frame False {
                n128 = local write "Raw"(w249) -> ()
              }
              frame True {
              }
            }
          }
        }
      }
      frame "---------- Core ----------" {
        n129 = call <vilib>:"Add State(s) to Queue__JKI_lib_State_Machine.vi"("State(s) in (\"\")"=w254) -> ("States Out"=w253:string)  [unwired: 14 in]
      }
      frame Default {
        w265 = 42 items=["No error", "Argument error", "Memory is full", "Out of zone", "End of file", "File already open", "Generic file I/O error", "File not found", "File permission error", "Disk is full", "Duplicate path", "Too many files open", "System feature not enabled", "Resource file not found", "Cannot add resource", "Resource not found", "Image not found", "Image memory error", "Pen does not exist", "Config type invalid", "Config token not found", "Config parse error", "Config memory error", "Bad external code format", "Bad external code offset", "External code not present", "Null window", "Destroy window error", "Null menu", "Print aborted", "Bad print record", "Print driver error", "Windows error during printing", "Memory error during printing", "Print dialog error", "Generic print error", "Invalid device refnum", "Device not found", "Device parameter error", "Device unit error", "Cannot open device", "Device call aborted", "Generic error", "Cancelled by user", "Object ID too low", "Object ID too high", "Object not in heap", "Unknown heap", "Unknown object (invalid DefProc)", "Unknown object (DefProc not in table)", "Message out of range", "Invalid (null) method", "Unknown message", "Manager call not supported", "Bad address", "Network operation in progress", "Network operation timed out", "Connection is busy", "Network attribute not supported", "Network error", "Address in use", "System out of memory", "Connection aborted", "Connection refused", "Not connected", "Already connected", "Connection closed", "Initialization error (interapplication manager)", "Bad occurrence", "Wait on unbound occurrence handler", "Occurrence queue overflow", "Datalog type conflict", "Unused", "Unrecognized type (interapplication manager)", "Memory corrupt", "Failed to make temporary DLL", "Old CIN version", "Drag socket not found", "Failed to load drop-object", "Failed to register OLE object", "Failed to release OLE object", "Format specifier type mismatch", "Unknown format specifier", "Too few format specifiers", "Too many format specifiers", "Scan failed", "Newer CIN version", "Error converting to variant", "Runtime menu error", "Password tampered", "Variant attribute not found", "Incompatible variant data type", "Event data is not available", "Event Store is not present", "Occurrence is not found", "Event Queue is not created", "Event info is not available", "Refnum passed is NULL", "Error retrieving Class GUID", "Error retrieving CoClass GUID", "Error retrieving TypeLib GUID.", "Bad built application magic bytes.", "Specific driver is different from the specific driver associated with the Logical Name.", "There is no session opened to the class driver.", "Max Error", "MAX - Error with config objects", "MAX - Error loading configuration", "MAX - Group not supported"]
        # "Current State"
        # "Do not delete, rename, or modify this frame.\n(this is used to capture unhandled states and typos)"
        # "Handle mistyped state name (developer tool)"
        n130 = Format Into String(format string="Software Exception: Unhandled State \"%s\"." ("message"), error in=w261, w256) -> (resulting string=w264:string, error out=w263:errorcluster)  [unwired: 1 in]
        n131 = call <vilib>:"Error Cluster From Error Code.vi"("show call chain? (False)"=TRUE, "error in (no error)"=w263, "error message (\"\")"=w264, "error code (0)"=w265) -> ("error out"=w262:errorcluster)  [unwired: 5 in]
        n132 = call <vilib>:"Add State(s) to Queue__JKI_lib_State_Machine.vi"("State(s) in (\"\")"=w260) -> ("States Out"=w259:string)  [unwired: 14 in]
      }
      frame "Initialize Core Data" {
        # "Do not delete, rename, or modify this frame.\n(this is used to determine panel behavior on exit)"
        # "originally closed?"
        # "exe?"
        # "If panel starts closed or is an EXE, then close it when we exit"
        n133 = property class="VI"() -> ("FP.State"=w270:T7)  [unwired: 2 in, 2 out]
        n134 = property class="App"() -> ("App.Kind"=w276:T8)  [unwired: 2 in, 2 out]
        n135 = control-ref of="Current VI Reference"() -> (w271:refnum<vi>)
        n136 = Equal?(x=w270, y=T7."Closed" ("Front Panel Window:State")) -> (x = y?=w268:bool)
        n137 = Equal?(x=w276, y=T8."Run Time System" ("Application:Kind")) -> (x = y?=w274:bool)
        n138 = Or(x=w268, y=w274) -> (x .or. y?=w272:bool)
        n139 = Bundle By Name(cluster=w273, "Core.Current VI Reference"=w271, "Core.Close Panel on Exit?"=w272) -> (w278:T12)
        n140 = call <vilib>:"Add State(s) to Queue__JKI_lib_State_Machine.vi"("State(s) in (\"\")"=w280) -> ("States Out"=w279:string)  [unwired: 14 in]
      }
      frame "Error Handler" {
        # "Unhandled Error -- Display it"
        # "Handle any errors here.\nYou can also output any states to clean-up after errors occur"
        # "Clear error"
        n141 = call <vilib>:"General Error Handler.vi"("error in (no error)"=w283) -> ()  [unwired: 10 in, 5 out]
        n142 = call <vilib>:"Add State(s) to Queue__JKI_lib_State_Machine.vi"("State(s) in Front (\"\")"="/* Post Error States", "State(s) in (\"\")"=w287) -> ("States Out"=w286:string)  [unwired: 13 in]
      }
      frame "Exit" {
        # "Do not put any code in this frame.\n(No errors that occur here will be handled.)"
        n143 = call <vilib>:"Add State(s) to Queue__JKI_lib_State_Machine.vi"("State(s) in (\"\")"=w293) -> ("States Out"=w292:string)  [unwired: 14 in]
      }
      frame "---------- Data ----------" {
        # "Do not put any code in this frame.\n(It is a separator no-op. You can make a copy of this frame to create a new Data frame)"
        n144 = call <vilib>:"Add State(s) to Queue__JKI_lib_State_Machine.vi"("State(s) in (\"\")"=w298) -> ("States Out"=w297:string)  [unwired: 14 in]
      }
      frame "Data: Initialize" {
        w307 = FALSE  # valid data
        w308 = "CALIBRATION_DATA"  # VAR
        w311 = T13 {"Current VI Reference"=refnum, "Close Panel on Exit?"=FALSE}  # Core
        n145 = call "MessageAMC_Create.vi"("reference in"=refnum<class "MessageAMC.lvclass"> refnum, "error in (no error)"=w303, "message queue name"="GUI_CALIBRATION_SENS") -> ("amc"=w304:refnum<class "MessageAMC.lvclass">, "error out"=w302:errorcluster)  [unwired: 15 in]
        n146 = control-ref of="Scales ref"() -> (w301:refnum<vi>)
        n147 = control-ref of="scale indx ref"() -> (w300:refnum<vi>)
        n148 = Bundle("Core"=w311, "CalibrationData"=T9 {"Channels"=[], "Scales"=[]}, "VAR"=w308, "valid data"=w307, "amc"=w304, "channel indx"="channel indx", "Scales ref"=w301, "scale indx ref"=w300) -> (w312:T12)  [unwired: 1 in]
      }
      frame "Data: Cleanup" {
        n149 = Unbundle By Name(w315) -> ("Core.Current VI Reference"=w318:refnum<vi>)
        n150 = Close Reference(reference=w318, error in (no error)=w317) -> (error out=w316:errorcluster)
        n151 = call <vilib>:"Add State(s) to Queue__JKI_lib_State_Machine.vi"("State(s) in (\"\")"=w320) -> ("States Out"=w319:string)  [unwired: 14 in]
      }
      frame "---------- Events ----------" {
        n152 = call <vilib>:"Add State(s) to Queue__JKI_lib_State_Machine.vi"("State(s) in (\"\")"=w325) -> ("States Out"=w324:string)  [unwired: 14 in]
      }
      frame "Events: Register" {
        n153 = call "Read stop event.vi"("GUI in"=w328) -> ("cmd event"=w326:refnum<user-event>, "stop event"=w327:refnum<user-event>)  [unwired: 8 in, 1 out]
        n154 = register-events(error in=w329, w327, w326) -> (reference out=w331:refnum<event-registration>, error out=w330:errorcluster)  [unwired: 1 in]
      }
      frame "Events: Unregister" {
        n155 = Unregister For Events(event registration refnum=w336, error in=w335) -> (error out=w334:errorcluster)
        n156 = call <vilib>:"Add State(s) to Queue__JKI_lib_State_Machine.vi"("State(s) in (\"\")"=w339) -> ("States Out"=w338:string)  [unwired: 14 in]
      }
      frame "---------- UI ----------" {
        # "Do not put any code in this frame.\n(It is a separator no-op. You can make a copy of this frame to create a new UI frame)"
        n157 = call <vilib>:"Add State(s) to Queue__JKI_lib_State_Machine.vi"("State(s) in (\"\")"=w344) -> ("States Out"=w343:string)  [unwired: 14 in]
      }
      frame "UI: Initialize" {
      }
      frame "UI: Cursor Set" {
        # "Argument"
        # "Set and Unset Cursor Busy.\n(Usage: \"UI: Cursor Set >> Busy|Idle\")"
        n158 = case shown="\"Idle\", Default" w350 {
          tunnel: w352 -> [w357 w359]
          tunnel: [w356 w358] -> w351
          frame "Idle", Default {
            n159 = call <vilib>:"Unset Busy.vi"("error in (no error)"=w357) -> ("error out"=w356:errorcluster)  [unwired: 10 in]
          }
          frame "Busy" {
            n160 = call <vilib>:"Set Busy.vi"("error in (no error)"=w359) -> ("error out"=w358:errorcluster)  [unwired: 9 in, 1 out]
          }
        }
        n161 = call <vilib>:"Add State(s) to Queue__JKI_lib_State_Machine.vi"("State(s) in (\"\")"=w355) -> ("States Out"=w354:string)  [unwired: 14 in]
      }
      frame "UI: Front Panel State" {
        # "Argument"
        # "Set Front Panel Open or Closed\n(Usage: \"UI: Front Panel State >> Open|Close\")"
        n162 = Unbundle By Name(w363) -> ("Core.Current VI Reference"=w362:refnum<vi>)
        n163 = case shown="\"Minimize\", \"Minimized\"" w361 {
          tunnel: w365 -> [w373 w388 w399 w412 w425]
          tunnel: [w375 w389 w401 w414 w427] -> w364
          tunnel: w362 -> [w374 w386 w400 w413 w426]
          frame "Open", "Standard", Default {
            w368 = T7."Standard" ("State")
            n164 = property class="VI"(reference=w374, error in=w373) -> (reference out=w371:refnum<vi>, error out=w372:errorcluster, "FP.State"=w370:T7)
            n165 = Not Equal?(x=w370, y=w368) -> (x != y?=w369:bool)
            n166 = case shown="True" w369 {
              tunnel: [w379 w381] -> w375
              tunnel: w372 -> [w378 w381]
              tunnel: w371 -> [w377 _]
              tunnel: w368 -> [w376 _]
              frame True {
                n167 = invoke class="VI" method="FP.Open"(reference=w377, error in=w378, "Activate"=TRUE, "State"=w376) -> (error out=w379:errorcluster)  [unwired: 1 in, 4 out]
              }
              frame False {
              }
            }
          }
          frame "Close", "Closed" {
            n168 = property class="VI"(reference=w386, error in=w388) -> (reference out=w385:refnum<vi>, error out=w387:errorcluster, "FP.State"=w383:T7)
            n169 = Not Equal?(x=w383, y=T7."Closed" ("Front Panel Window:State")) -> (x != y?=w382:bool)
            n170 = case shown="True" w382 {
              tunnel: [w390 w393] -> w389
              tunnel: w387 -> [w390 w392]
              tunnel: w385 -> [_ w391]
              frame False {
              }
              frame True {
                n171 = invoke class="VI" method="FP.Close"(reference=w391, error in=w392) -> (error out=w393:errorcluster)  [unwired: 1 in, 2 out]
              }
            }
          }
          frame "Hidden", "Hide" {
            w394 = T7."Hidden" ("State")
            n172 = property class="VI"(reference=w400, error in=w399) -> (reference out=w397:refnum<vi>, error out=w398:errorcluster, "FP.State"=w396:T7)
            n173 = Not Equal?(x=w396, y=w394) -> (x != y?=w395:bool)
            n174 = case shown="True" w395 {
              tunnel: [w405 w406] -> w401
              tunnel: w398 -> [w404 w406]
              tunnel: w397 -> [w403 _]
              tunnel: w394 -> [w402 _]
              frame True {
                n175 = invoke class="VI" method="FP.Open"(reference=w403, error in=w404, "State"=w402) -> (error out=w405:errorcluster)  [unwired: 2 in, 4 out]
              }
              frame False {
              }
            }
          }
          frame "Minimize", "Minimized" {
            w407 = T7."Minimized" ("State")
            n176 = property class="VI"(reference=w413, error in=w412) -> (reference out=w410:refnum<vi>, error out=w411:errorcluster, "FP.State"=w409:T7)
            n177 = Not Equal?(x=w409, y=w407) -> (x != y?=w408:bool)
            n178 = case shown="True" w408 {
              tunnel: [w418 w419] -> w414
              tunnel: w411 -> [w417 w419]
              tunnel: w410 -> [w416 _]
              tunnel: w407 -> [w415 _]
              frame True {
                n179 = invoke class="VI" method="FP.Open"(reference=w416, error in=w417, "State"=w415) -> (error out=w418:errorcluster)  [unwired: 2 in, 4 out]
              }
              frame False {
              }
            }
          }
          frame "Maximize", "Maximized" {
            w420 = T7."Maximized" ("State")
            n180 = property class="VI"(reference=w426, error in=w425) -> (reference out=w423:refnum<vi>, error out=w424:errorcluster, "FP.State"=w422:T7)
            n181 = Not Equal?(x=w422, y=w420) -> (x != y?=w421:bool)
            n182 = case shown="True" w421 {
              tunnel: [w431 w432] -> w427
              tunnel: w424 -> [w430 w432]
              tunnel: w423 -> [w429 _]
              tunnel: w420 -> [w428 _]
              frame True {
                n183 = invoke class="VI" method="FP.Open"(reference=w429, error in=w430, "State"=w428) -> (error out=w431:errorcluster)  [unwired: 2 in, 4 out]
              }
              frame False {
              }
            }
          }
        }
        n184 = call <vilib>:"Add State(s) to Queue__JKI_lib_State_Machine.vi"("State(s) in (\"\")"=w367) -> ("States Out"=w366:string)  [unwired: 14 in]
      }
      frame "---------- Macro ----------" {
        # "Do not put any code in this frame.\n(It is a separator no-op. You can make a copy of this frame to create a new Macro frame)"
        n185 = call <vilib>:"Add State(s) to Queue__JKI_lib_State_Machine.vi"("State(s) in (\"\")"=w437) -> ("States Out"=w436:string)  [unwired: 14 in]
      }
      frame "Macro: Initialize" {
        n186 = call <vilib>:"Add State(s) to Queue__JKI_lib_State_Machine.vi"("State(s) in Front (\"\")"="Data: Initialize\nInitialize Core Data\nEvents: Register\nUI: Initialize\n// UI: Front Panel State >> Open\n\n\n", "State(s) in (\"\")"=w443) -> ("States Out"=w442:string)  [unwired: 13 in]
      }
      frame "Macro: Write" {
        n187 = call <vilib>:"Add State(s) to Queue__JKI_lib_State_Machine.vi"("State(s) in Front (\"\")"="Action: Write Config", "State(s) in (\"\")"=w449) -> ("States Out"=w448:string)  [unwired: 13 in]
      }
      frame "Macro: Read" {
        n188 = call <vilib>:"Add State(s) to Queue__JKI_lib_State_Machine.vi"("State(s) in Front (\"\")"="Action: Read Config\nAction: Update Controls", "State(s) in (\"\")"=w455) -> ("States Out"=w454:string)  [unwired: 13 in]
      }
      frame "Macro: Exit" {
        # "Exit Macro\n(This is called once, when the VI exits)"
        n189 = Unbundle By Name(w464) -> ("Core.Close Panel on Exit?"=w463:bool)
        n190 = Select(t="UI: Front Panel State >> Close", s=w463, f="") -> (s? t:f=w460:string)
        n191 = call <vilib>:"Add State(s) to Queue__JKI_lib_State_Machine.vi"("State(s) in Front (\"\")"="Macro: Write", "State(s) in (\"\")"=w460, "State(s) at Back (\"\")"="Data: Cleanup\nEvents: Unregister\nExit") -> ("States Out"=w458:string)  [unwired: 12 in]
        n192 = call <vilib>:"Add State(s) to Queue__JKI_lib_State_Machine.vi"("State(s) in Front (\"\")"=w458, "State(s) in (\"\")"=w467) -> ("States Out"=w466:string)  [unwired: 13 in]
      }
      frame "---------- Action ----------" {
      }
      frame "Action: Read Config" {
        n193 = call "Read SVW.vi"("GUI in"=w479) -> ("SharedVariableWrapper.lvclass"=w478:refnum<class "SharedVariableWrapper.lvclass">)  [unwired: 10 in]
        n194 = Unbundle By Name(w481) -> ("VAR"=w480:string)
        n195 = in-place {
          in-place-border: [w492] -> w482
          in-place-border: w480 -> [w491]
          in-place-border: w478 -> [w490]
          in-place-border: w477 -> [w487]
          in-place-border: [w486] -> w473
          n196 = in-place-cluster #15(w481) -> ("CalibrationData"=w493:T9)  [unwired: 1 out]
          n197 = call "Read.vim"("SharedVariableWrapper in"=w490, "name"=w491, "DataType"=w493, "error in (no error)"=w487) -> ("connected"=w486:bool, "data out"=w489:T9, "error out"=w492:errorcluster)  [unwired: 5 in, 4 out]
          n198 = call "Check Channels Name.vi"("data in"=w489) -> ("data out"=w488:T9)  [unwired: 14 in]
          n199 = in-place-cluster #15("CalibrationData"=w488, "valid data"=w486) -> (w483:T12)
        }
        n200 = case shown="False" w473 {
          tunnel: ["Action: Read Config" ("State(s) in Front (\"\")") _] -> w474
          frame False {
          }
          frame True {
          }
        }
        n201 = call <vilib>:"Clear Errors.vi"("error in (no error)"=w482) -> ("error out"=w472:errorcluster)  [unwired: 5 in, 1 out]
        n202 = call <vilib>:"Add State(s) to Queue__jki_lib_state_machine.vi"("State(s) in Front (\"\")"=w474, "State(s) in (\"\")"=w475) -> ("States Out"=w476:string)  [unwired: 13 in]
      }
      frame "Action: Write Config" {
        n203 = Unbundle By Name(w497) -> ("valid data"=w498:bool)
        n204 = call "Read SVW.vi"("GUI in"=w496) -> ("SharedVariableWrapper.lvclass"=w495:refnum<class "SharedVariableWrapper.lvclass">)  [unwired: 10 in]
        n205 = case shown="True" w498 {
          tunnel: w497 -> [_ w507]
          tunnel: w495 -> [_ w505]
          tunnel: w494 -> [_ w504]
          frame False {
          }
          frame True {
            n206 = call "ReadConfig.vi"("SharedVariableWrapper in"=w505, "error in"=w504) -> ("config"=w503:T14, "error out"=w501:errorcluster)  [unwired: 11 in, 1 out]
            n207 = Unbundle By Name(w507) -> ("amc"=w513:refnum<class "MessageAMC.lvclass">, "CalibrationData"=w506:T9)
            n208 = Unbundle By Name(w503) -> ("ip"=w502:string)
            n209 = call "SendNetworkVariant.vi"("reference in"=w513, "receiver process"="STAND", "receiver host"=w502, "receiver port (0)"=u16 54321, "name"="SET_CALIBRATION_DATA", "data"=w506, "timeout (25000 ms)"=1000, "error in (no error)"=w501) -> ("error out"=w510:errorcluster)  [unwired: 5 in, 2 out]
            n210 = call <vilib>:"Simple Error Handler.vi"("error in (no error)"=w510) -> ()  [unwired: 4 in, 5 out]
          }
        }
      }
      frame "Action: Update Controls" {
        n211 = Unbundle By Name(w523) -> ("CalibrationData.Channels"=w544:T10[], "channel indx"=w535:T3, "Scales ref"=w534:refnum<vi>, "scale indx ref"=w532:refnum<vi>, "CalibrationData.Scales"=w528:T5[])
        n212 = Index Array(array=w544, index=w535) -> (element=w538:T10)
        n213 = Unbundle By Name(w523) -> ("CalibrationData.Scales"=w521:T5[], "CalibrationData.Channels"=w524:T10[], "channel indx"=w525:T3)
        n214 = Index Array(array=T11 [] ("Strings And Values []")) -> (element=w530:cluster{"String":string, "Value":u16})  [unwired: 1 in]
        n215 = for {
          tunnel: w544 -> [w561] mode=indexing
          tunnel: [w558] -> w514 mode=indexing
          n216 = Unbundle By Name(w561) -> ("Name"=w560:string, "ScaleIndex"=w559:u32)
          n217 = Bundle("Name"=w560, "ScaleIndex"=w559) -> (w558:cluster{"Name":string, "ScaleIndex":u32})  [unwired: 1 in]
        }
        n218 = for {
          tunnel: w528 -> [w557] mode=indexing
          tunnel: [w555] -> w533 mode=indexing
          tunnel: w530 -> [w556]
          tunnel: [w554] -> w529 mode=indexing
          n219 = Unbundle By Name(w557) -> ("Name"=w555:string, "index"=w553:i32)
          n220 = Bundle By Name(cluster=w556, "String"=w555, "Value"=w553) -> (w554:cluster{"String":string, "Value":u16})
        }
        n221 = Unbundle By Name(w538) -> ("AI Ranges"=w537:T4)
        n222 = control-ref of="Gauge"() -> (w536:refnum<vi>)
        n223 = Index Array(array=w524, index=w525) -> (element=w526:T10)
        n224 = Unbundle By Name(w526) -> ("ScaleIndex"=w527:u32)
        n225 = local write "AI Ranges"(w537) -> ()
        n226 = call "Set Color Zones.vim"("reference"=w536, "AI Ranges"=w537) -> ()  [unwired: 13 in, 1 out]
        n227 = for {
          tunnel: w521 -> [w552] mode=indexing
          tunnel: w527 -> [w551]
          tunnel: [w549] -> _
          tunnel: [w548] -> w522
          i -> [w548]
          stop <- w549 stop-if-true
          n228 = Unbundle By Name(w552) -> ("index"=w550:i32)
          n229 = Equal?(x=w550, y=w551) -> (x = y?=w549:bool)
        }
        n230 = local write "channels"(w514) -> ()
        n231 = property class="LstBox (strict)"(reference=w534, "Item Names"=w533) -> ()  [unwired: 1 in, 2 out]
        n232 = property class="Ring (strict)"(reference=w532, "StringsAndValues[]"=w529) -> ()  [unwired: 1 in, 2 out]
        n233 = Index Array(array=w521, index=w522) -> (element=w520:T5)
        n234 = Unbundle By Name(w520) -> ("X"=w518:dbl[], "Y"=w517:dbl[], "Name"=w515:string)
        n235 = property on="XY Graph - Dark" class="XYGraph (strict)"("Caption.Text"=w515) -> ()  [unwired: 2 in, 2 out]
        n236 = Number To Fractional String(number=w517, precision (6)=i16 3) -> (F-format string=w542:string[])  [unwired: 2 in]
        n237 = Number To Fractional String(number=w518, precision (6)=i16 3) -> (F-format string=w541:string[])  [unwired: 2 in]
        n238 = Bundle("X"=w518, "Y"=w517) -> (→"XY Graph - Dark":cluster{"X":dbl[], "Y":dbl[]})  [unwired: 1 in]
        n239 = Build Array(w541, w542) -> (w519:string[][])
        n240 = Transpose 2D Array(2D array=w519) -> (transposed array=w543:string[][])
        n241 = property on="data" class="MCListbox (strict)"("ItemNames"=w543) -> ()  [unwired: 2 in, 2 out]
      }
    }
  }
  "error out" <- w6
